vi "gyro app -- V1.vi"() -> ()   [LabVIEW 2020]
uses:
  launch items list.ctl
  pll internal user event action.ctl
  que event bag action.ctl
  server talkto message type.ctl
  server talkback message type.ctl
  cursor action.ctl
panel:
  in  "Main":enum32{"all", "other"}(tab)
  in  "exit!":bool=TRUE
  in  "procs":cluster{"item":T1, "gear":bool}[](array[cluster])=[{"item"=enum."source", "gear"=FALSE}, {"item"=enum."fitter", "gear"=FALSE}, {"item"=enum."sweeper engine", "gear"=FALSE}, {"item"=enum."sweeper monitor", "gear"=FALSE}, {"item"=enum."pll engine", "gear"=FALSE}, {"item"=enum."pll monitor", "gear"=FALSE}]
  in  "Cluster":cluster{"item":T1, "gear":bool}={"item"=enum."sweeper engine", "gear"=FALSE}
  in  "launch items":T1=enum."sweeper engine"
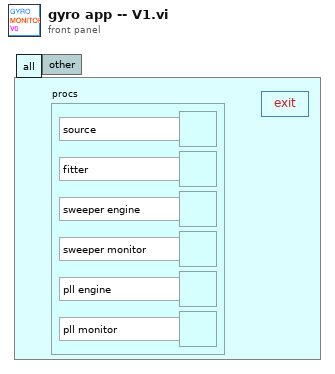
[diagram p1: front panel]
types:
  T1 = typedef "launch items list.ctl" = enum16{"source", "pll engine", "pll monitor", "sweeper engine", "sweeper monitor", "fitter"}
  T2 = typedef "pll internal user event action.ctl" = enum16{"gear pll engine", "start pll async", "stop pll async", "toggle pll async", "gear sweeper", "start sweeper", "stop sweeper", "toggle sweeper", "accept frequency", "reset lorentzian", "accept lorentzian", "update cursors", "pause pll", "unpause pll", "void", "exit", "gear sweeper monitor", "gear sweeper engine", "gear fitter", "gear sourcer", "gear pll monitor"}
  T3 = typedef "que event bag action.ctl" = enum16{"check", "add", "init", "keys", "values"}
  T4 = typedef "server talkback message type.ctl" = cluster{"message":enum16{"new", "void"}}
  T5 = typedef "server talkto message type.ctl" = cluster{"message":enum16{"stop", "start", "update pars", "update request", "new", "launch", "exit", "get", "reset", "pause", "unpause"}}
  T6 = typedef "server talk-to-back pair.ctl" = cluster{"talkback event":refnum<user-event>, "talkto event":refnum<user-event>}
  T7 = typedef "cursor action.ctl" = enum16{"range", "read", "write", "check", "zoom out", "smart zoom out", "zoom to aspect ratio 1", "zoom to win", "zoom out 20%", "zoom in 20%", "-empty", "smart zoom out&aspect", "move range left 20%", "move range right 20%", "move range up 20%", "move range down 20%", "zoom to X win", "zoom to Y win", "zoom out X", "zoom out Y", "zoom in X", "zoom in Y", "check plot scale"}
  T8 = enum32{"Invalid", "Standard", "Closed", "Hidden", "Minimized", "Maximized"}
  T9 = typedef "eventvkey.ctl" = enum16{"ASCII", "Enter", "Return", "Shift", "Ctrl", "Alt", "Cmd", "Opt", "Caps", "NumLock", "Clear", "Break", "Up", "Down", "Left", "Right", "Insert", "Delete", "Home", "End", "PageUp", "PageDown", "Escape", "Help", "Pause", "ScrollLock", "F1", "F2", "F3", "F4", "F5", "F6", "F7", "F8", "F9", "F10", "F11", "F12", "F13", "F14", "F15", "F16", "F17", "F18", "F19", "F20", "F21", "F22", "F23", "F24", "Play", "VolumeUp", "VolumeDown", "Mute", "Two Byte Char"}
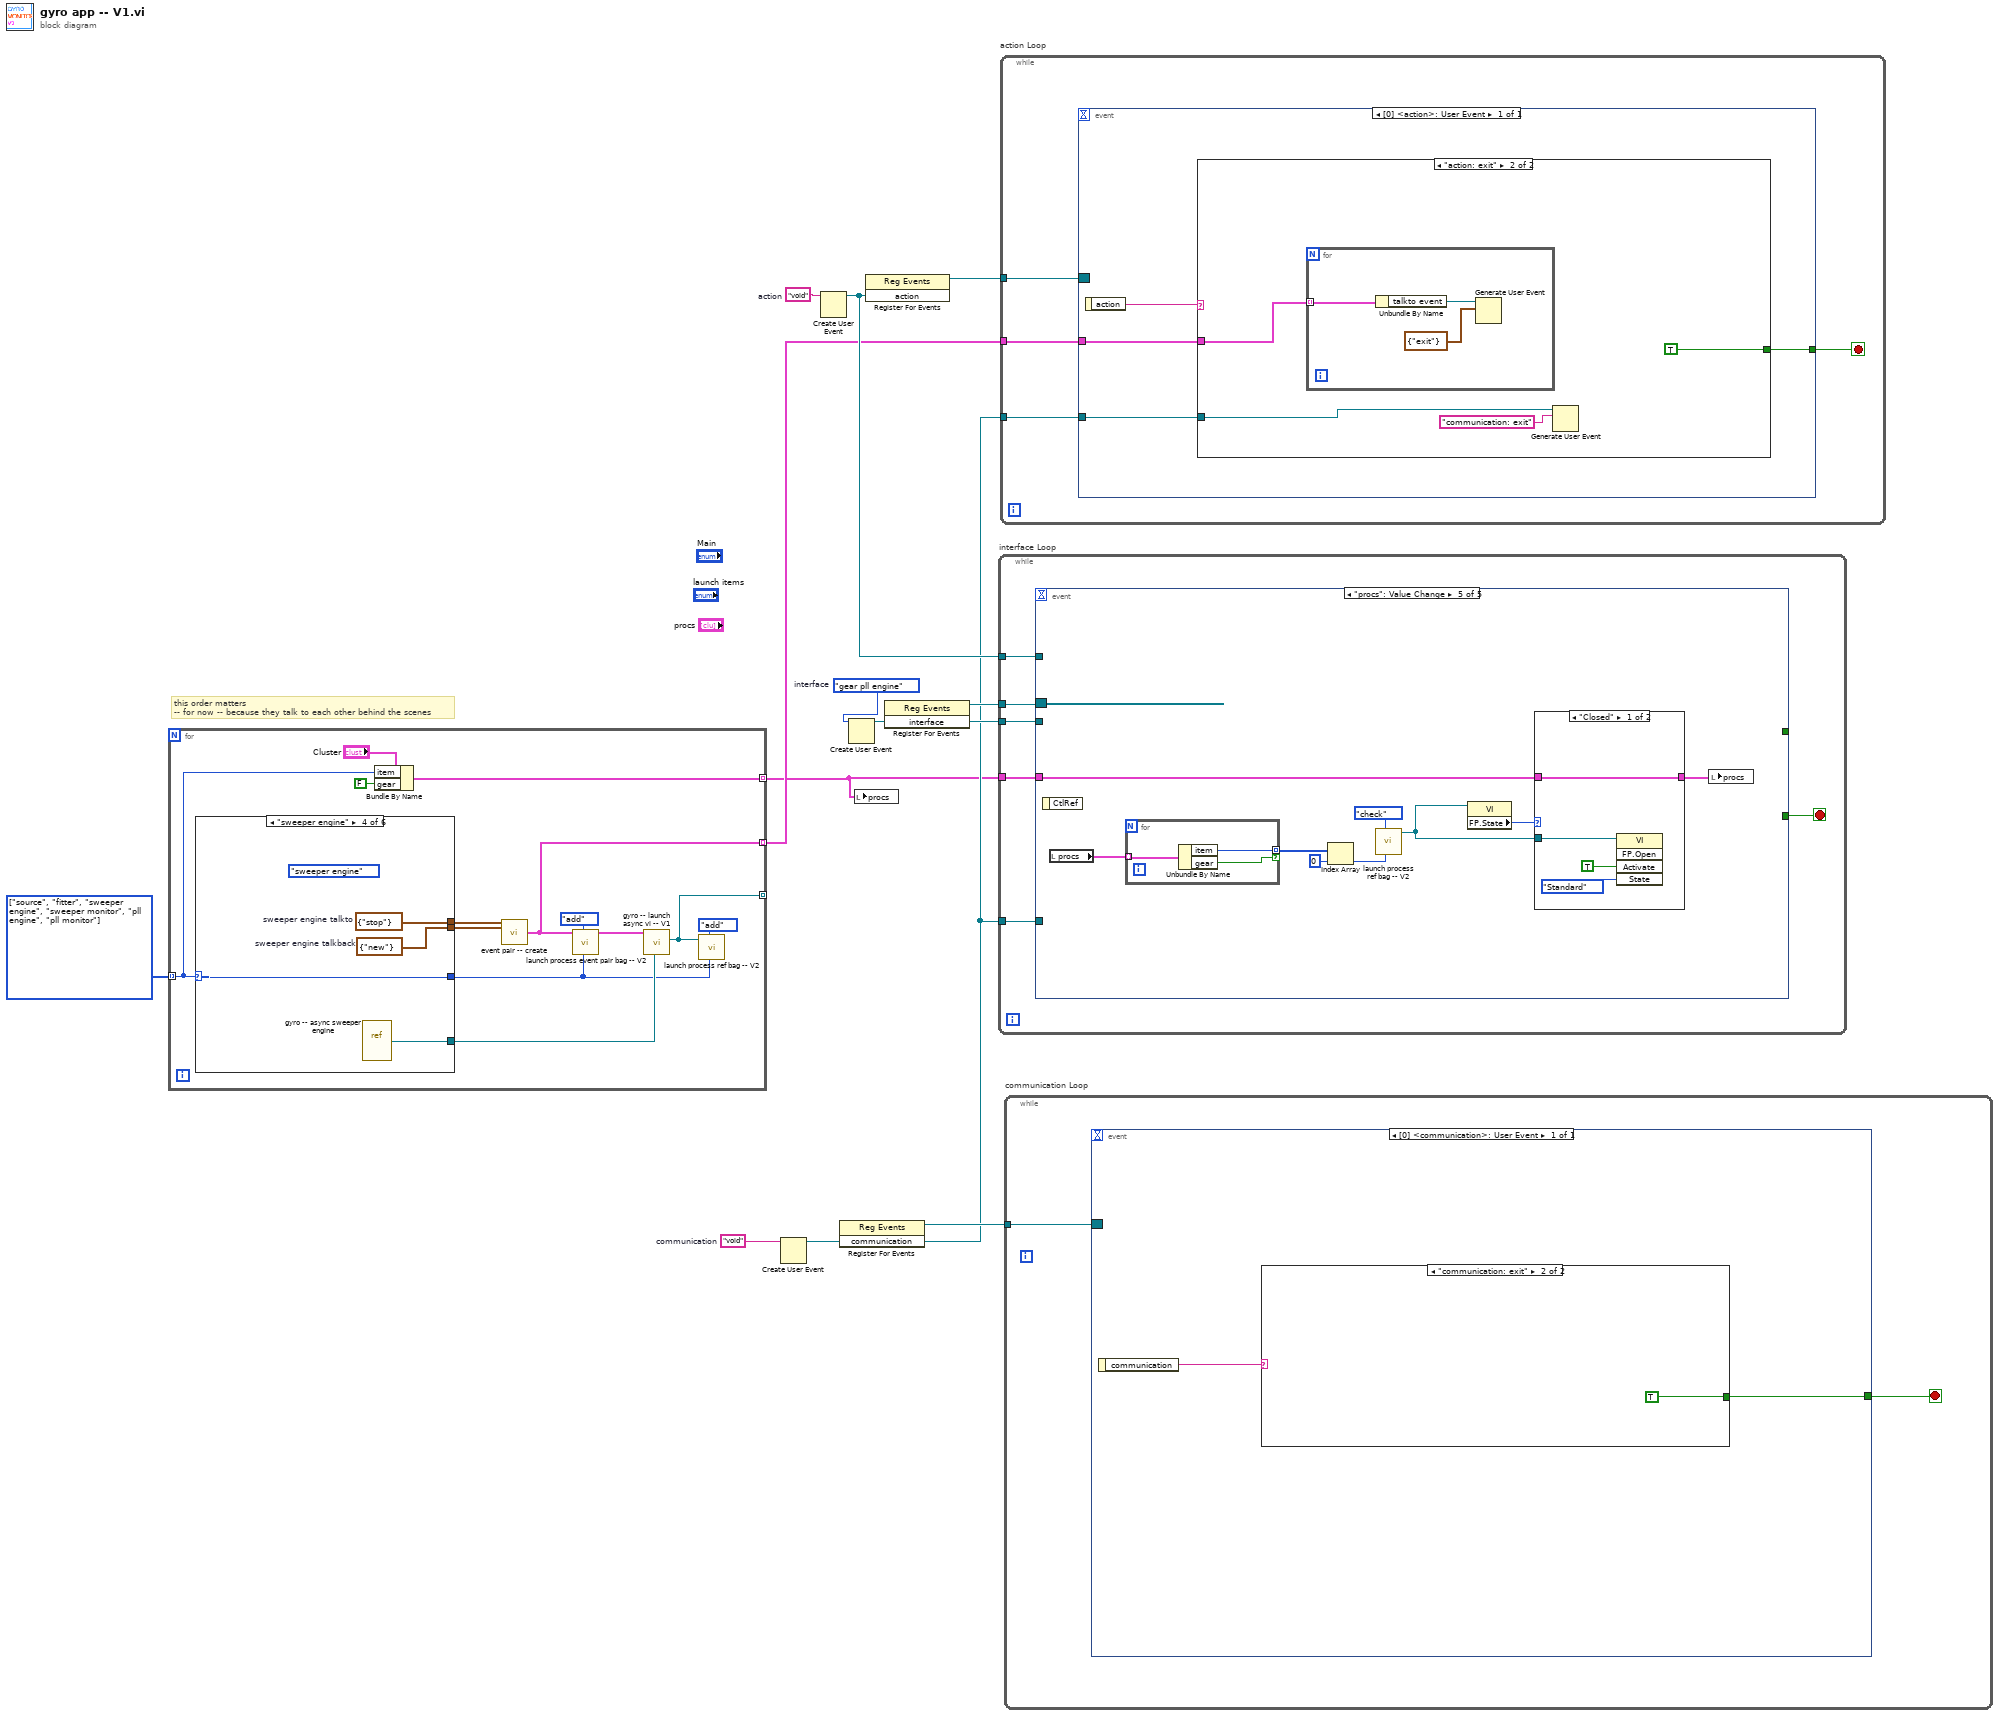
[diagram p0: block diagram]
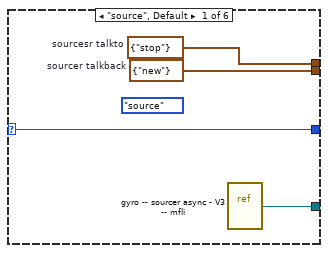
[diagram p2: hidden frame]
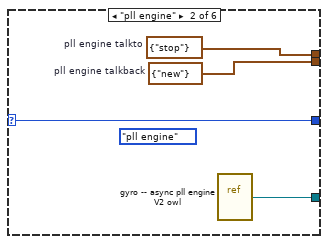
[diagram p3: hidden frame]
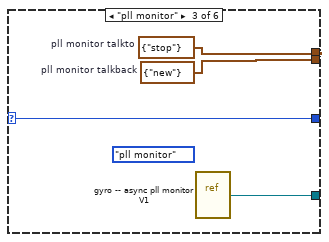
[diagram p4: hidden frame]
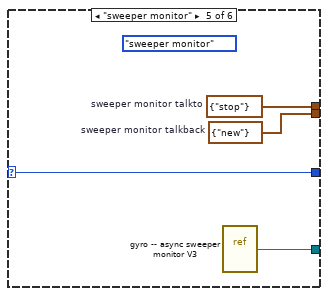
[diagram p5: hidden frame]
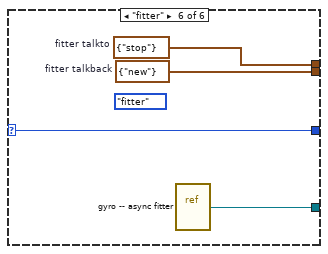
[diagram p6: hidden frame]
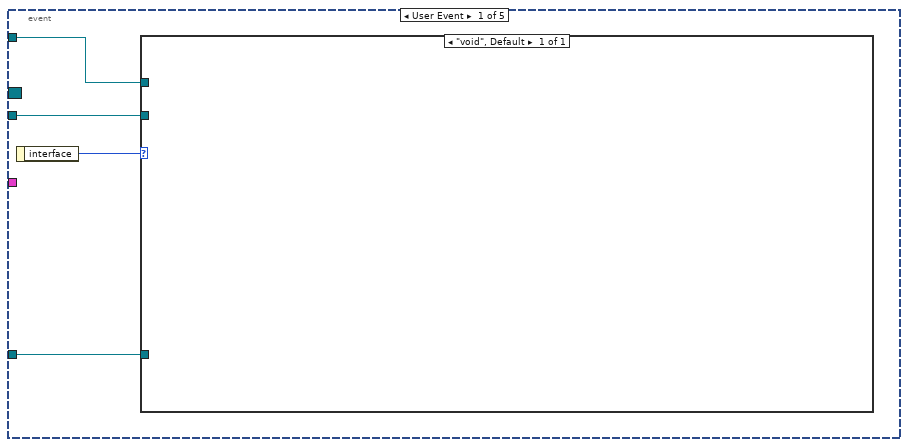
[diagram p9: hidden frame]
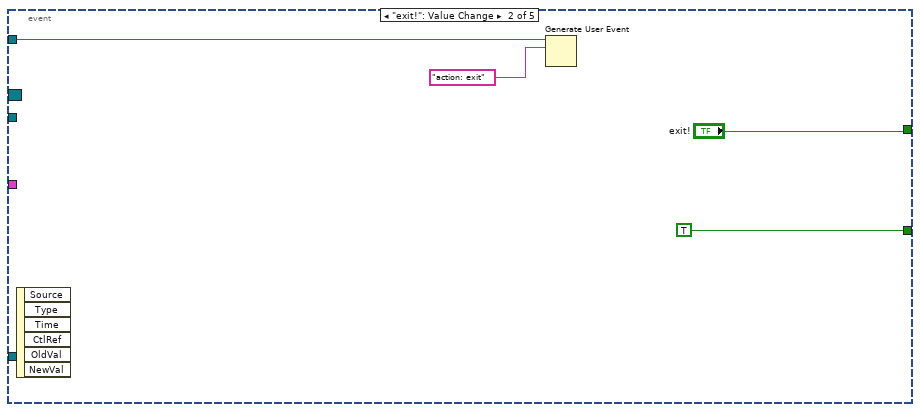
[diagram p10: hidden frame]
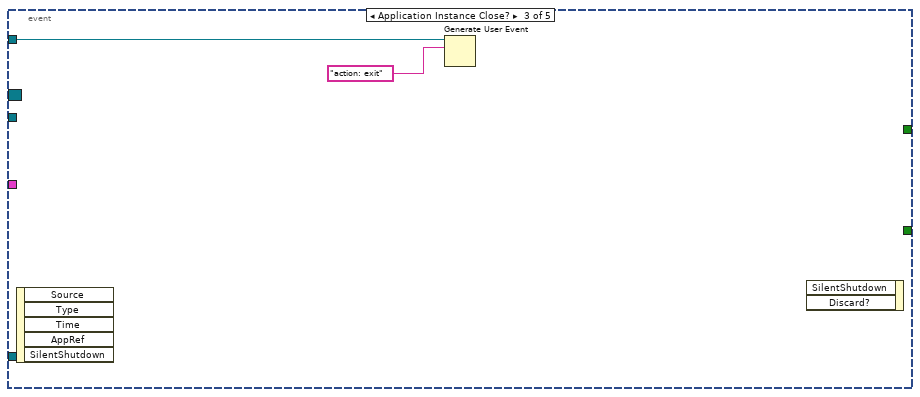
[diagram p11: hidden frame]
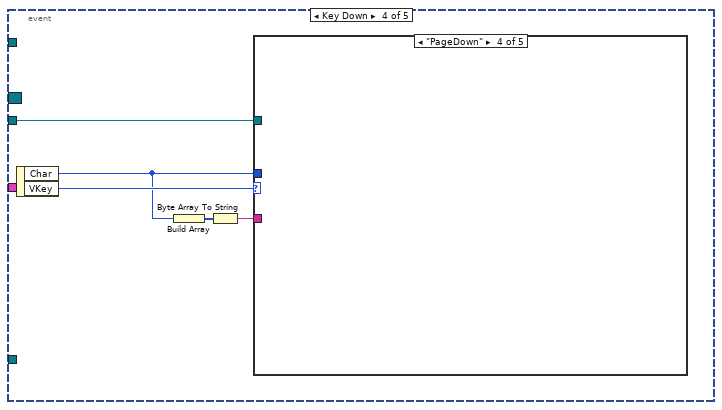
[diagram p12: hidden frame]
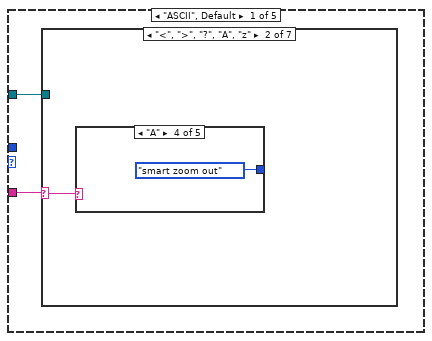
[diagram p13: hidden frame]
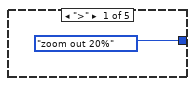
[diagram p15: hidden frame]
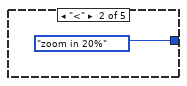
[diagram p16: hidden frame]
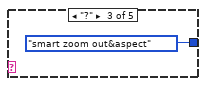
[diagram p17: hidden frame]
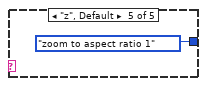
[diagram p18: hidden frame]
diagram:
  w2 = T1[] [enum."source", enum."fitter", enum."sweeper engine", enum."sweeper monitor", enum."pll engine", enum."pll monitor"] items=["source", "pll engine", "pll monitor", "sweeper engine", "sweeper monitor", "fitter"]
  w5 = "void"  # communication
  w8 = "void"  # action
  w10 = pll_internal_user_event_action."gear pll engine"  # interface
  # "this order matters\n-- for now -- because they talk to each other behind the scenes"
  n1 = for {
    tunnel: w2 -> [w14] mode=indexing
    tunnel: [w20] -> w4 mode=indexing
    tunnel: [w17] -> _ mode=indexing
    tunnel: [w13] -> w1 mode=indexing
    n2 = case shown="\"sweeper engine\"" w14 {
      selector: w14 -> [w29 w33 w37 w38 w43 w49]
      tunnel: [w27 w31 w35 w41 w45 w48] -> w22
      tunnel: [w26 w30 w34 w40 w44 w47] -> w21
      tunnel: [w29 w33 w37 w38 w43 w49] -> w18
      tunnel: [w28 w32 w36 w39 w42 w46] -> w19
      frame "source", Default {
        (unwired) launch_items_list."source" ("launch items")
        w26 = T4 {"message"=enum."new"}  # sourcer talkback
        w27 = T5 {"message"=enum."stop"}  # sourcesr talkto
        n3 = vi-ref "gyro -- sourcer async - V3 -- mfli.vi"() -> (w28:refnum<vi>)
      }
      frame "pll engine" {
        (unwired) launch_items_list."pll engine" ("launch items")
        w30 = T4 {"message"=enum."new"}  # pll engine talkback
        w31 = T5 {"message"=enum."stop"}  # pll engine talkto
        n4 = vi-ref "gyro -- async pll engine V2 owl.vi"() -> (w32:refnum<vi>)
      }
      frame "pll monitor" {
        (unwired) launch_items_list."pll monitor" ("launch items")
        w34 = T4 {"message"=enum."new"}  # pll monitor talkback
        w35 = T5 {"message"=enum."stop"}  # pll monitor talkto
        n5 = vi-ref "gyro -- async pll monitor V1.vi"() -> (w36:refnum<vi>)
      }
      frame "sweeper engine" {
        (unwired) launch_items_list."sweeper engine" ("launch items")
        w40 = T4 {"message"=enum."new"}  # sweeper engine talkback
        w41 = T5 {"message"=enum."stop"}  # sweeper engine talkto
        n6 = vi-ref "gyro -- async sweeper engine.vi"() -> (w39:refnum<vi>)
      }
      frame "sweeper monitor" {
        (unwired) launch_items_list."sweeper monitor" ("launch items")
        w44 = T4 {"message"=enum."new"}  # sweeper monitor talkback
        w45 = T5 {"message"=enum."stop"}  # sweeper monitor talkto
        n7 = vi-ref "gyro -- async sweeper monitor V3.vi"() -> (w42:refnum<vi>)
      }
      frame "fitter" {
        (unwired) launch_items_list."fitter" ("launch items")
        w47 = T4 {"message"=enum."new"}  # fitter talkback
        w48 = T5 {"message"=enum."stop"}  # fitter talkto
        n8 = vi-ref "gyro -- async fitter.vi"() -> (w46:refnum<vi>)
      }
    }
    n9 = Bundle By Name(cluster="Cluster", "item"=w14, "gear"=FALSE) -> (w13:cluster{"item":T1, "gear":bool})
    n10 = call "event pair -- create.vi"("talkto"=w22, "talkback"=w21) -> ("even pair out"=w20:T6)  [unwired: 11 in, 2 out]
    n11 = call "launch process event pair bag -- V2.vi"("launch item"=w18, "bag action"=que_event_bag_action."add", "event pair IN"=w20) -> ("event pair OUT"=w25:T6)  [unwired: 6 in, 2 out]
    n12 = call "gyro -- launch async vi -- V1.vi"("VI Refnum"=w19, "pll event pair IN"=w25) -> ("reference out"=w17:refnum<vi>)  [unwired: 8 in, 1 out]
    n13 = call "launch process ref bag -- V2.vi"("launch item"=w18, "bag action"=que_event_bag_action."add", "process ref IN"=w17) -> ()  [unwired: 6 in, 3 out]
  }
  n14 = Create User Event(user event datatype=w5) -> (user event=w3:refnum<user-event>)  [unwired: 1 in, 1 out]
  n15 = Create User Event(user event datatype=w8) -> (user event=w6:refnum<user-event>)  [unwired: 1 in, 1 out]
  n16 = register-events(w3) -> (reference out=w11:refnum<event-registration>)  [unwired: 2 in, 1 out]
  n17 = Create User Event(user event datatype=w10) -> (user event=w9:refnum<user-event>)  [unwired: 1 in, 1 out]
  n18 = local write "procs"(w1) -> ()
  n19 = register-events(w6) -> (reference out=w7:refnum<event-registration>)  [unwired: 2 in, 1 out]
  n20 = register-events(w9) -> (reference out=w12:refnum<event-registration>)  [unwired: 2 in, 1 out]
  n21 = while "interface Loop" {
    tunnel: w12 -> [w55]
    tunnel: w9 -> [w54]
    tunnel: w6 -> [w52]
    tunnel: w3 -> [w51]
    tunnel: w1 -> [w50]
    stop <- w53 stop-if-true
    n22 = event shown="[4] \"procs\": Value Change" {
      selector: w55 -> [_ _ _ _ _]
      dyn-events: _ -> [_ _ _ _ _]
      timeout: _ -> [_ _ _ _ _]
      tunnel: [_ "exit!" _ _ _] -> _
      tunnel: w54 -> [w58 _ _ w66 _]
      tunnel: [_ TRUE _ _ _] -> w53
      tunnel: w52 -> [w57 w61 w64 _ _]
      tunnel: w51 -> [w56 _ _ _ _]
      tunnel: w50 -> [_ _ _ _ w84]
      event User Event {
        n23 = event-data() -> ("interface"=w59:T2)  [unwired: 1 in]
        n24 = case shown="\"void\", Default" w59 {
          tunnel: w58 -> [_]
          tunnel: w57 -> [_]
          tunnel: w56 -> [_]
          frame "void", Default {
          }
        }
      }
      event "exit!": Value Change {
        n25 = event-data() -> ()  [unwired: 1 in, 6 out]
        n26 = Generate User Event(user event=w61, event data cluster="action: exit" ("event data")) -> ()  [unwired: 2 in, 2 out]
      }
      event Application Instance Close? {
        n27 = event-data() -> ()  [unwired: 1 in, 5 out]
        n28 = Generate User Event(user event=w64, event data cluster="action: exit" ("event data")) -> ()  [unwired: 2 in, 2 out]
        n29 = event-data() -> ()  [unwired: 3 in, 1 out]
      }
      event Key Down {
        n30 = event-data() -> ("Char"=w68:i16, "VKey"=w70:T9)  [unwired: 1 in]
        n31 = Build Array(w68) -> (w69:i16[])
        n32 = Byte Array To String(unsigned byte array=w69) -> (string=w67:string)
        n33 = case shown="\"PageDown\"" w70 {
          selector: w70 -> [_ _ _ _ w79]
          tunnel: w68 -> [_ _ _ _ _]
          tunnel: w67 -> [w72 _ _ _ _]
          tunnel: w66 -> [w71 _ _ _ _]
          frame "ASCII", Default {
            n34 = case shown="\"<\", \">\", \"?\", \"A\", \"z\"" w72 {
              selector: w72 -> [_ w73 _ _ _ _ _]
              tunnel: w71 -> [_ _ _ _ _ _ _]
              frame "0", Default {
              }
              frame "<", ">", "?", "A", "z" {
                n35 = case shown="\"A\"" w73 {
                  tunnel: [cursor_action."zoom out 20%" ("cursor action") cursor_action."zoom in 20%" ("cursor action") cursor_action."smart zoom out&aspect" ("cursor action") cursor_action."smart zoom out" ("cursor action") cursor_action."zoom to aspect ratio 1" ("cursor action")] -> _
                  frame ">" {
                  }
                  frame "<" {
                  }
                  frame "?" {
                  }
                  frame "A" {
                  }
                  frame "z", Default {
                  }
                }
              }
              frame "r" {
              }
              frame "'", ";", "[", "]", "{", "}" {
              }
              frame "@" {
              }
              frame "#" {
              }
              frame "q" {
              }
            }
          }
          frame "Escape" {
          }
          frame "PageUp" {
          }
          frame "PageDown" {
          }
          frame "Up".."Right" {
            n36 = case shown="\"Down\"" w79 {
              tunnel: [cursor_action."move range right 20%" ("cursor action") cursor_action."move range left 20%" ("cursor action") cursor_action."move range up 20%" ("cursor action") cursor_action."move range down 20%" ("cursor action")] -> _
              frame "Right", Default {
              }
              frame "Left" {
              }
              frame "Up" {
              }
              frame "Down" {
              }
            }
          }
        }
      }
      event "procs": Value Change {
        n37 = event-data() -> ()  [unwired: 1 in, 1 out]
        n38 = local read "procs"() -> (w88:cluster{"item":T1, "gear":bool}[])
        n39 = for {
          tunnel: w88 -> [w95] mode=indexing
          tunnel: [w93] -> w87 mode=indexing if=w94
          n40 = Unbundle By Name(w95) -> ("item"=w93:T1, "gear"=w94:bool)
        }
        n41 = Index Array(array=w87, index=0) -> (element=w89:T1)
        n42 = call "launch process ref bag -- V2.vi"("launch item"=w89, "bag action"=que_event_bag_action."check") -> ("process ref OUT"=w90:refnum<vi>)  [unwired: 7 in, 2 out]
        n43 = property class="VI"(reference=w90) -> ("FP.State"=w92:T8)  [unwired: 1 in, 2 out]
        n44 = case shown="\"Closed\"" w92 {
          tunnel: w90 -> [w99 w101]
          tunnel: [w96 w100] -> w85
          tunnel: w84 -> [w96 w100]
          frame "Closed" {
            n45 = invoke class="VI" method="FP.Open"(reference=w99, "Activate"=TRUE ("Activate?"), "State"=T8."Standard" ("Front Panel Window:State")) -> ()  [unwired: 2 in, 5 out]
          }
          frame "Standard", Default {
            n46 = invoke class="VI" method="FP.Close"(reference=w101) -> ()  [unwired: 2 in, 3 out]
          }
        }
        n47 = local write "procs"(w85) -> ()
      }
    }
  }
  n48 = while "action Loop" {
    tunnel: w7 -> [w105]
    tunnel: w4 -> [w103]
    tunnel: w3 -> [w102]
    stop <- w104 stop-if-true
    n49 = event shown="[0] <action>: User Event" {
      selector: w105 -> [_]
      dyn-events: _ -> [_]
      timeout: _ -> [_]
      tunnel: [w108] -> w104
      tunnel: w103 -> [w107]
      tunnel: w102 -> [w106]
      event User Event {
        n50 = event-data() -> ("action"=w109:string)  [unwired: 1 in]
        n51 = case shown="\"action: exit\"" w109 {
          tunnel: [_ TRUE] -> w108
          tunnel: w107 -> [_ w112]
          tunnel: w106 -> [_ w110]
          frame "action: void", Default {
          }
          frame "action: exit" {
            n52 = for {
              tunnel: w112 -> [w114] mode=indexing
              n53 = Unbundle By Name(w114) -> ("talkto event"=w115:refnum<user-event>)
              n54 = Generate User Event(user event=w115, event data cluster=T5 {"message"=enum."exit"} ("event data")) -> ()  [unwired: 2 in, 2 out]
            }
            n55 = Generate User Event(user event=w110, event data cluster="communication: exit" ("event data")) -> ()  [unwired: 2 in, 2 out]
          }
        }
      }
    }
  }
  n56 = while "communication Loop" {
    tunnel: w11 -> [w118]
    stop <- w117 stop-if-true
    n57 = event shown="[0] <communication>: User Event" {
      selector: w118 -> [_]
      dyn-events: _ -> [_]
      timeout: _ -> [_]
      tunnel: [w119] -> w117
      event User Event {
        n58 = event-data() -> ("communication"=w120:string)  [unwired: 1 in]
        n59 = case shown="\"communication: exit\"" w120 {
          tunnel: [_ TRUE] -> w119
          frame "void", Default {
          }
          frame "communication: exit" {
          }
        }
      }
    }
  }
